vi "PicoScope5000aExampleRapidBlockBulkOverlapped.vi"() -> ()   [LabVIEW 2010]
uses:
  shared/PicoBuffers.ctl
  <vilib>/Waveform/DWDTOps.llb/DWDT Analog to Digital.vi
  PicoScope5000aLib/PicoScope5000aAnalogChannelSettings.ctl
  shared/Segment Range.ctl
  shared/Buffer and Transfer Settings.ctl
  shared/Acquisition Settings.ctl
  shared/nSegments.ctl
  PicoScope5000aLib/PicoScope5000aDigitalChannelSettings.ctl
panel:
  in  "Channel B Settings":T1={"Enabled"=FALSE, "Coupling"=1, "Range"=6, "Analogue Offset"=0.0, "Bandwidth Limit"=0} {"Bandwidth Limit" items=["Full", "20MHz"]; "Range" items=["10 mV", "20 mV", "50 mV", "100 mV", "200 mV", "500 mV", "1 V", "2 V", "5 V", "10 V", "20 V"]; "Coupling" items=["AC", "DC"]}
  out "Total Requested Samples":u64
  out "overflow":i16[](array[numeric]) format="%06b"
  in  "Port 0 Settings":T2={"Enabled"=FALSE, "Logic Level"=9830} {"Logic Level" items=["1.5V TTL"=9830, "2.5V CMOS"=16383]}
  in  "Channel A Settings":T1={"Enabled"=TRUE, "Coupling"=1, "Range"=6, "Analogue Offset"=0.0, "Bandwidth Limit"=0} {"Bandwidth Limit" items=["Full", "20MHz"]; "Range" items=["10 mV", "20 mV", "50 mV", "100 mV", "200 mV", "500 mV", "1 V", "2 V", "5 V", "10 V", "20 V"]; "Coupling" items=["AC", "DC"]}
  in  "Trigger Settings":T3={"Trigger Enabled"=FALSE, "Trigger Source"=enum."Channel A", "Trigger Threshold (volts)"=0.0, "Trigger Direction"=2, "Trigger Delay (samples)"=0, "Auto Trigger Time (ms)"=1000} {"Trigger Direction" items=["Rising"=2, "Falling"=3]}
  out "USB 3.0 device on non-USB 3.0 Port":bool
  out "USB Powered":bool=TRUE
  out "Device Info":T4={"Driver Version"="2.1.104.3324", "USB Version"="2.0", "Hardware"="1", "Variant"="5244A", "Batch and Serial"="CQ178/007", "Cal Date"="11Jun13", "Kernel Version"="1.0", "Digital HW Version"="1", "Analogue HW Version"="1", "MSO"=FALSE, "Number of channels"=2}
  out "Trigger Offsets":cluster{"Samples":u64, "Time (seconds)":sgl}[](array[cluster]) {"Time (seconds)" format="%#_5p"}
  in  "Stop Display":bool
  out "Capture Complete":bool
  in  "Run":bool
  in  "Display Buffer Index":i32
  in  "Segment Range":T5={"fromSegmentIndex"=0, "toSegmentIndex"=9} {"toSegmentIndex" format="%.4p"; "fromSegmentIndex" format="%.4p"}
  in  "nSegments":T6=10 format="%.4p"
  out "error out":errorcluster
  in  "Data file":path=path "PicoScope5000aExampleRapidBlock ChA Data"
  in  "Buffer and Transfer Settings":T7={"startIndex"=0, "Samples"=5000000, "Down Sample Ratio"=2, "Down-Sample Mode"=1} {"Down-Sample Mode" items=["RAW none"=2147483648, "None"=0, "Aggregate"=1, "Decimate"=2, "Average"=4]; "Down Sample Ratio" step=1; "Samples" format="%_6p"}
  in  "Acquisition Settings":T8={"preTriggerSamples"=0, "postTriggerSamples"=5000000, "timebase"=5} {"postTriggerSamples" format="%_6p"; "preTriggerSamples" format="%_6p"}
  out "Properties Panel":T9={"Sample Frequency"=41666668.0, "Sample Rate"=2.4000000209412065e-08, "Max Samples Available"=26843008, "Number of Samples"=0, "Total Capture Time (sec) "=0.0, "Max Total Capture Time Available (sec)"=0.6442322134971619} {"Max Total Capture Time Available (sec)" format="%.3p"; "Sample Frequency" format="%.6p"; "Sample Rate" format="%.3p"; "Max Samples Available" format="%_6p"; "Total Capture Time (sec)" format="%.3p"}
  out "Port 0":digitalwaveform(graph)={"t0"=timestamp(0 s since 1904-01-01), "dt"=8e-09, "Y"={"transitions"=[], "data"=[]}}
  in  "stop":bool
  out "Analog Channels":cluster{i32, sgl, "Data":dbl[]}[](graph)
  in  "Resolution":u32(ring) items=["8-bit"=0, "12-bit"=1, "14-bit"=2, "15-bit"=3, "16-bit"=4, "10-bit"=10]
  in  "Serial Number":string
  in  "Use Serial Number":bool
  in  "error in (no error)":errorcluster
  # "Number of\nSegments to Capture"
  # "Bit 0 = ChA"
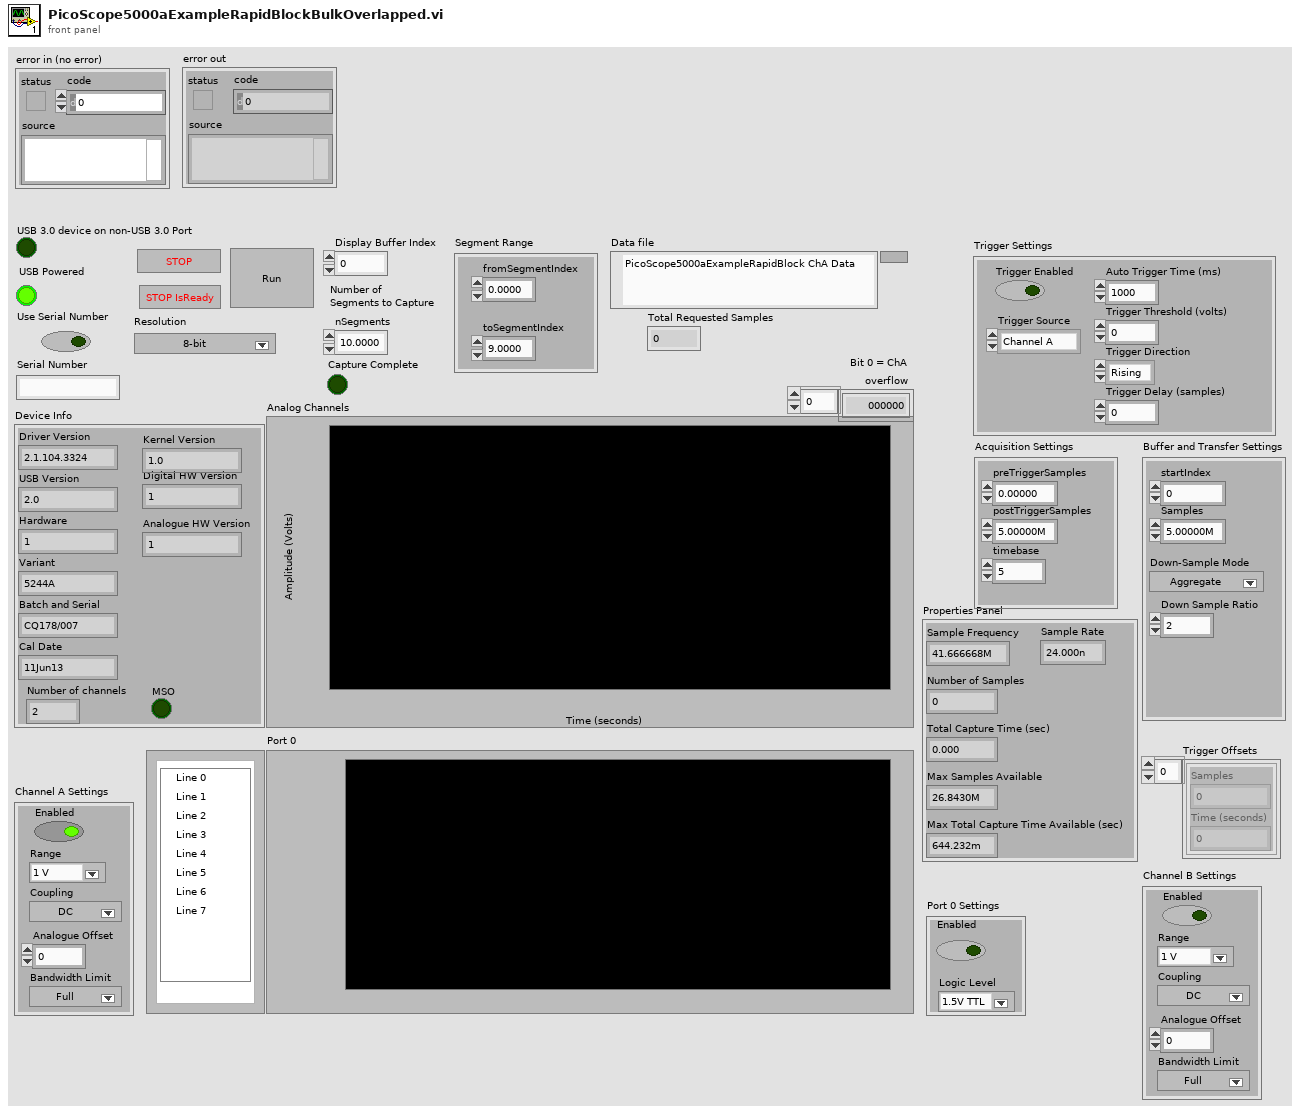
[diagram p1: front panel]
types:
  T1 = typedef "PicoScope5000aAnalogChannelSettings.ctl" = cluster{"Enabled":bool, "Coupling":i16, "Range":u16, "Analogue Offset":sgl, "Bandwidth Limit":u32}
  T2 = typedef "PicoScope5000aDigitalChannelSettings.ctl" = cluster{"Enabled":bool, "Logic Level":i16}
  T3 = cluster{"Trigger Enabled":bool, "Trigger Source":enum16{"Channel A", "Channel B", "Channel C", "Channel D", "Ext."}, "Trigger Threshold (volts)":dbl, "Trigger Direction":u16, "Trigger Delay (samples)":u32, "Auto Trigger Time (ms)":i16}
  T4 = cluster{"Driver Version":string, "USB Version":string, "Hardware":string, "Variant":string, "Batch and Serial":string, "Cal Date":string, "Kernel Version":string, "Digital HW Version":string, "Analogue HW Version":string, "MSO":bool, "Number of channels":i16}
  T5 = typedef "Segment Range.ctl" = cluster{"fromSegmentIndex":u64, "toSegmentIndex":u64}
  T6 = typedef "nSegments.ctl" = u64
  T7 = typedef "Buffer and Transfer Settings.ctl" = cluster{"startIndex":u64, "Samples":u64, "Down Sample Ratio":u64, "Down-Sample Mode":u32}
  T8 = typedef "Acquisition Settings.ctl" = cluster{"preTriggerSamples":u64, "postTriggerSamples":u64, "timebase":u32}
  T9 = cluster{"Sample Frequency":dbl, "Sample Rate":dbl, "Max Samples Available":u64, "Number of Samples":u64, "Total Capture Time (sec) ":dbl, "Max Total Capture Time Available (sec)":dbl}
  T10 = enum16{"open", "open or create", "create or replace", "create", "open (read-only)"}
  T11 = cluster{"Channel A Buffer":i16[], "Channel B Buffer":i16[], "Channel C Buffer":i16[], "Channel D Buffer":i16[], "Channel E Buffer":i16[], "Channel F Buffer":i16[], "Channel G Buffer":i16[], "Channel H Buffer":i16[], "Port 0 Buffer":i16[], "Port 1 Buffer":i16[]}[]
  T12 = typedef "PicoBuffers.ctl" = cluster{"Max Buffer Pointers":u64[][][], "Min Buffer Pointers":u64[][][], "StreamingDataInfo":cluster{"Channel":u32, "Down-Sample Mode":u32, "PICO_DATA_TYPE":enum32{"PICO_INT8_T", "PICO_INT16_T", "PICO_INT32_T", "PICO_UINT32_T", "PICO_INT64_T", ""}, "Samples":i32, "bufferIndex":u64, "startIndex":i32, "overflow":i16}[][]}
  T13 = cluster{"Sample Frequency":sgl, "Sample Rate":sgl, "Max Samples Available":i32, "Number of Samples":u32, "Total Capture Time (sec) ":sgl, "Max Total Capture Time Available (sec)":sgl}
  T14 = cluster{"Channel A Buffer":i16[], "Channel B Buffer":i16[], "Channel C Buffer":i16[], "Channel D Buffer":i16[], "Channel E Buffer":i16[], "Channel F Buffer":i16[], "Channel G Buffer":i16[], "Channel H Buffer":i16[], "Port 0 Buffer":i16[], "Port 1 Buffer":i16[]}
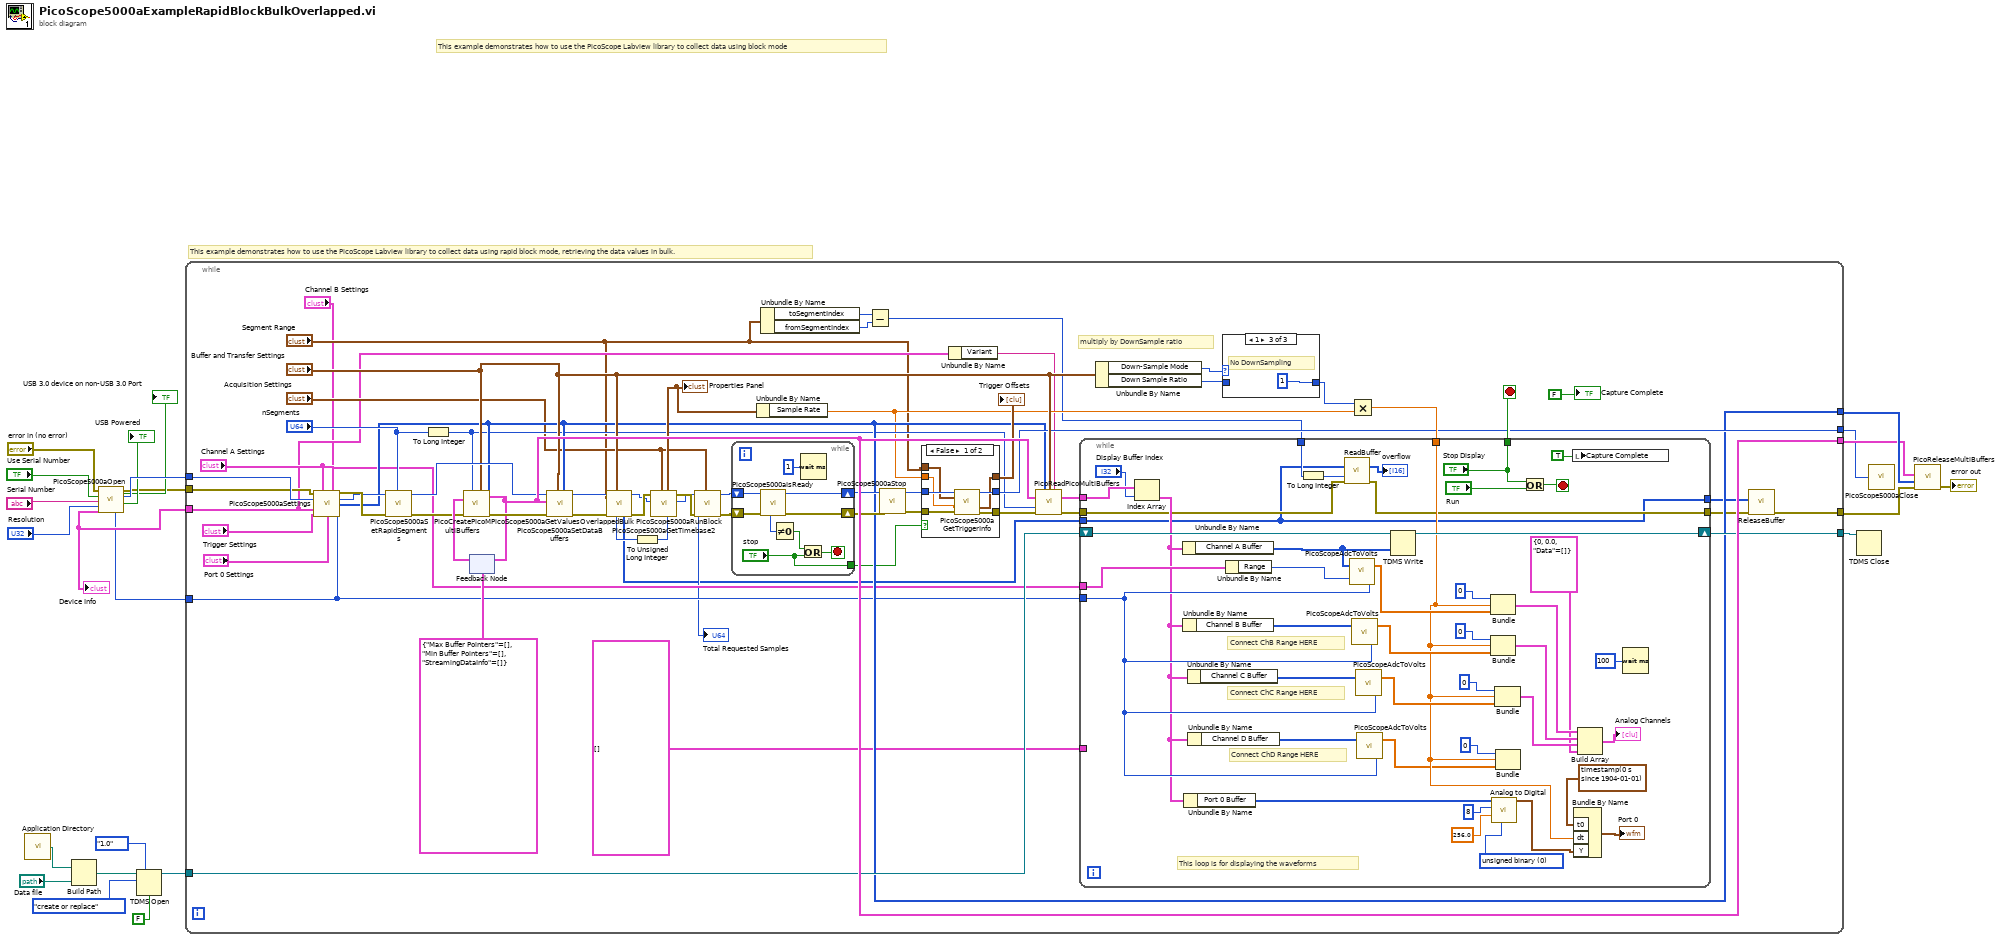
[diagram p0: block diagram]
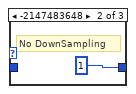
[diagram p4: hidden frame]
diagram:
  # "This example demonstrates how to use the PicoScope Labview library to collect data using rapid block mode, retrieving the data values in bulk."
  # "This example demonstrates how to use the PicoScope Labview library to collect data using block mode"
  n1 = call <vilib>:"Application Directory.vi"() -> ("Application Directory"=w14:path)
  n2 = Build Path(base path=w14, name or relative path="Data file") -> (appended path=w15:path)
  n3 = call "PicoScope5000aOpen.vi"("Serial Number"="Serial Number", "Resolution"="Resolution", "Use Serial Number"="Use Serial Number", "error in (no error)"="error in (no error)") -> ("USB Powered"=→"USB Powered":bool, "handle"=w23:i16, "error out"=w2:errorcluster, "Max ADC value"=w5:i16, "USB 3.0 device on non-USB 3.0 Port"=→"USB 3.0 device on non-USB 3.0 Port":bool, "Device Info"=w6:T4)  [unwired: 2 in]
  "Device Info" <- w6
  n4 = TDMS Open(6:FALSE ("disable buffering? (T)"), 7:enum16{"1.0", "2.0"}."1.0" ("file format version (2.0)"), 10:T10."create or replace" ("operation (0:open)"), 11:w15) -> (3:w12:refnum<k34>)  [unwired: 2 in, 1 out]
  n5 = while {
    tunnel: w23 -> [w49]
    tunnel: w5 -> [w41]
    tunnel: [w61] -> w20
    tunnel: [w46] -> w22
    tunnel: [w82] -> w21
    tunnel: [w81] -> w13
    tunnel: w12 -> [w80]
    tunnel: w6 -> [w37]
    tunnel: w2 -> [w48]
    tunnel: [w32] -> w1
    stop <- w65 stop-if-true
    # "multiply by DownSample ratio"
    n6 = call "PicoScope5000aSettings.vi"("error in"=w48, "Channel A Settings"="Channel A Settings", "Port 0 Settings"="Port 0 Settings", "Channel B Settings"="Channel B Settings", "handle in"=w49, "Device Info"=w37, "Trigger Settings"="Trigger Settings", "Max ADC value"=w41) -> ("error out"=w51:errorcluster, "handle out"=w50:i16, "enabled array"=w46:i16[])  [unwired: 5 in]
    n7 = call "PicoScope5000aSetRapidSegments.vi"("nSegments"="nSegments", "error in (no error)"=w51, "handle in"=w50) -> ("error out"=w79:errorcluster, "handle out"=w78:i16)  [unwired: 6 in, 1 out]
    n8 = To Long Integer(number="nSegments") -> (32bit integer=w44:i32)
    n9 = feedback #1(T12 {"Max Buffer Pointers"=[], "Min Buffer Pointers"=[], "StreamingDataInfo"=[]} ("Data Pointers")) -> (w84:T12)
    n10 = call "PicoCreatePicoMultiBuffers.vi"("Number of Buffers"=w44, "Buffer and Transfer Settings"="Buffer and Transfer Settings", "enabled array"=w46, "Data Pointers In"=w84, "error in (no error)"=w79) -> ("Data Pointers"=w82:T12, "error out"=w83:errorcluster)  [unwired: 9 in]
    n11 = feedback-in #1(w82) -> ()
    n12 = call "PicoScope5000aSetDataBuffers.vi"("enabled array"=w46, "Buffer and Transfer Settings"="Buffer and Transfer Settings", "error in (no error)"=w83, "Data Pointers In"=w82, "handle in"=w78) -> ("error out"=w77:errorcluster, "handle out"=w76:i16)  [unwired: 5 in]
    n13 = call "PicoScope5000aGetValuesOverlappedBulk.vi"("Segment Range"="Segment Range", "Buffer and Transfer Settings"="Buffer and Transfer Settings", "error in (no error)"=w77, "handle in"=w76) -> ("error out"=w55:errorcluster, "handle out"=w54:i16, "Pointer to Overflow"=w30:u64[], "noOfSamples"=w35:u64)  [unwired: 4 in]
    n14 = To Unsigned Long Integer(number=w35) -> (unsigned 32bit integer=w34:u32)
    n15 = call "PicoScope5000aGetTimebase2.vi"("Number of Samples"=w34, "Acquisition Settings"="Acquisition Settings", "handle in"=w54, "error in (no error)"=w55) -> ("handle out"=w52:i16, "error out"=w53:errorcluster, "Properties Panel"=w71:T13)  [unwired: 5 in]
    "Properties Panel" <- w71
    n16 = call "PicoScope5000aRunBlock.vi"("Acquisition Settings"="Acquisition Settings", "error in (no error)"=w53, "handle in"=w52) -> ("error out"=w68:errorcluster, "handle out"=w67:i16, "Total Requested Samples"=→"Total Requested Samples":u64)  [unwired: 5 in, 1 out]
    n17 = while {
      shift-right: [w146] -> w59
      shift-left: w68 -> [w147]
      shift-right: [w145] -> w56
      shift-left: w67 -> [w144]
      tunnel: ["stop"] -> w40
      stop <- w140 stop-if-true
      n18 = call "PicoScope5000aIsReady.vi"("error in (no error)"=w147, "handle in"=w144) -> ("error out"=w146:errorcluster, "handle out"=w145:i16, "ready"=w142:i16)  [unwired: 7 in]
      n19 = Not Equal To 0?(x=w142) -> (x != 0?=w141:bool)
      n20 = Wait (ms)(milliseconds to wait=u32 1) -> ()  [unwired: 1 out]
      n21 = Or(x=w141, y="stop") -> (x .or. y?=w140:bool)
    }
    n22 = Unbundle By Name(w71) -> ("Sample Rate"=w39:sgl)
    n23 = Unbundle By Name("Segment Range") -> ("toSegmentIndex"=w28:u64, "fromSegmentIndex"=w27:u64)
    n24 = Subtract(x=w28, y=w27) -> (x-y=w25:u64)
    n25 = call "PicoScope5000aStop.vi"("error in (no error)"=w59, "handle in"=w56) -> ("error out"=w58:errorcluster, "handle out"=w57:i16)  [unwired: 8 in]
    n26 = case shown="False" w40 {
      tunnel: [w92 w93] -> w62
      tunnel: [w91 w94] -> w61
      tunnel: [w90 _] -> w60
      tunnel: w58 -> [w89 w93]
      tunnel: w57 -> [w88 w94]
      tunnel: "Segment Range" -> [w87 _]
      tunnel: w39 -> [w86 _]
      frame False {
        n27 = call "PicoScope5000aGetTriggerInfo.vi"("handle in"=w88, "Rapid Block Acquisition Settings"=w87, "Sample Rate"=w86, "error in"=w89) -> ("handle out"=w91:i16, "Trigger Offsets"=w90:cluster{u64, sgl}[], "error out"=w92:errorcluster)  [unwired: 8 in, 1 out]
      }
      frame True {
      }
    }
    "Trigger Offsets" <- w60
    n28 = Unbundle By Name(w37) -> ("Variant"=w38:string)
    n29 = call "PicoReadPicoMultiBuffers.vi"("enabled array"=w46, "Buffer and Transfer Settings"="Buffer and Transfer Settings", "Variant"=w38, "Data Pointers"=w82, "No of Buffers"=w44, "error in (no error)"=w62) -> ("MultiBuffers (Max or non-aggregated)"=w74:T11, "error out"=w66:errorcluster)  [unwired: 7 in, 1 out]
    n30 = Unbundle By Name("Buffer and Transfer Settings") -> ("Down-Sample Mode"=w72:u32, "Down Sample Ratio"=w73:u64)
    n31 = case shown="1" w72 {
      tunnel: [w148 u64 1 ("Down Sample Ratio") u64 1 ("Down Sample Ratio")] -> w69
      tunnel: w73 -> [w148 _ _]
      frame Default {
      }
      frame -2147483648 {
        # "No DownSampling"
      }
      frame 1 {
        # "No DownSampling"
      }
    }
    n32 = Multiply(x=w69, y=w39) -> (x*y=w70:sgl)
    n33 = while {
      tunnel: w41 -> [w109]
      tunnel: "Channel A Settings" -> [w138]
      tunnel: w74 -> [w108]
      tunnel: w70 -> [w110]
      shift-right: [w137] -> w81
      shift-left: w80 -> [w136]
      tunnel: [w98] -> w31
      tunnel: w66 -> [w99]
      tunnel: ["Stop Display"] -> w65
      tunnel: T11 [] ("array") -> [_]
      tunnel: w30 -> [w95]
      tunnel: [w95] -> w29
      tunnel: w25 -> [w96]
      stop <- w118 stop-if-true
      w127 = u16 0 items=["unsigned binary", "offset binary", "2's complement"] ("data format (offset binary)")
      # "This loop is for displaying the waveforms"
      # "Connect ChB Range HERE"
      # "Connect ChD Range HERE"
      # "Connect ChC Range HERE"
      n34 = Index Array(array=w108, index="Display Buffer Index") -> (element=w101:T14)
      n35 = Unbundle By Name(w101) -> ("Channel A Buffer"=w102:i16[])
      n36 = Unbundle By Name(w101) -> ("Channel B Buffer"=w133:i16[])
      n37 = Unbundle By Name(w101) -> ("Port 0 Buffer"=w125:i16[])
      n38 = Unbundle By Name(w101) -> ("Channel C Buffer"=w114:i16[])
      n39 = Unbundle By Name(w101) -> ("Channel D Buffer"=w106:i16[])
      n40 = Unbundle By Name(w138) -> ("Range"=w104:u16)
      n41 = To Long Integer(number=w96) -> (32bit integer=w100:i32)
      n42 = call "ReadBuffer.vi"("Pointer and BufferSize"=w95, "Buffer size"=w100, "error in (no error)"=w99) -> ("Output Array"=→"overflow":i16[], "error out"=w98:errorcluster)  [unwired: 11 in]
      n43 = call "PicoScopeAdcToVolts.vi"("Max_adc"=w109, "Range Index"=w104, "Data"=w102) -> ("Data"=w121:dbl[])
      n44 = call "PicoScopeAdcToVolts.vi"("Max_adc"=w109, "Data"=w133) -> ("Data"=w132:dbl[])  [unwired: 1 in]
      n45 = call "PicoScopeAdcToVolts.vi"("Max_adc"=w109, "Data"=w114) -> ("Data"=w113:dbl[])  [unwired: 1 in]
      n46 = call "PicoScopeAdcToVolts.vi"("Max_adc"=w109, "Data"=w106) -> ("Data"=w105:dbl[])  [unwired: 1 in]
      n47 = TDMS Write(0:w136, 9:w102) -> (4:w137:refnum<k34>)  [unwired: 4 in, 3 out]
      n48 = Bundle(0, w110, "Data"=w121) -> (w131:cluster{i32, sgl, "Data":dbl[]})  [unwired: 1 in]
      n49 = Bundle(0, w110, "Data"=w132) -> (w130:cluster{i32, sgl, "Data":dbl[]})  [unwired: 1 in]
      n50 = call-poly <vilib>:"Analog to Digital.vi"("data format (offset binary)"=w127, "full-scale range (pk-pk)"=256.0, "resolution (16 bit)"=8, "analog waveform"=w125) -> ("digital waveform"=w122:digitalwaveform)  [unwired: 4 in, 3 out]
      n51 = Bundle(0, w110, "Data"=w113) -> (w112:cluster{i32, sgl, "Data":dbl[]})  [unwired: 1 in]
      n52 = Bundle(0, w110, "Data"=w105) -> ()  [unwired: 1 in, 1 out]
      n53 = Or(x="Stop Display", y="Run") -> (x .or. y?=w118:bool)
      n54 = local write "Capture Complete"(TRUE ("Capture Complete")) -> ()
      n55 = Bundle By Name("t0"=timestamp(0 s since 1904-01-01), "dt"=w110, "Y"=w122) -> (→"Port 0":digitalwaveform)  [unwired: 1 in]
      n56 = Build Array(w131, w130, w112, cluster{i32, sgl, "Data":dbl[]} {0, 0.0, "Data"=[]} ("element")) -> (→"Analog Channels":cluster{i32, sgl, "Data":dbl[]}[])
      n57 = Wait (ms)(milliseconds to wait=u32 100) -> ()  [unwired: 1 out]
    }
    n58 = call "ReleaseBuffer.vi"("error in (no error)"=w31, "Pointer and BufferSize"=w29) -> ("error out"=w32:errorcluster)  [unwired: 9 in]
    "Capture Complete" <- FALSE ("Capture Complete")
  }
  n59 = TDMS Close(11:w13) -> ()  [unwired: 1 in, 2 out]
  n60 = call "PicoScope5000aClose.vi"("handle"=w20) -> ()
  n61 = call "PicoReleaseMultiBuffers.vi"("error in (no error)"=w1, "Enabled array"=w22, "Data Pointers"=w21) -> ("error out"=→"error out":errorcluster)  [unwired: 8 in]
